vi "Get-date-string.vi"() -> (3 "Date string":string)   [LabVIEW 2013, in "HardwareCharacterization.lvlib" / "HC-Main.lvclass"]
uses:
  HC-Main.lvclass
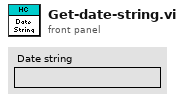
[diagram p1: front panel]
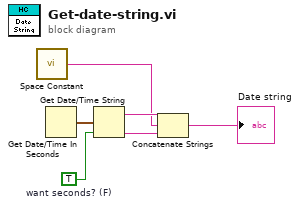
[diagram p0: block diagram]
diagram:
  w1 = TRUE  # want seconds? (F)
  n1 = call <vilib>:"Space Constant.vi"() -> ("String"=w2:string)
  n2 = Get Date/Time In Seconds() -> (seconds since 1Jan1904=w4:timestamp)
  n3 = Get Date/Time String(seconds (now)=w4, want seconds? (F)=w1) -> (date string=w5:string, time string=w3:string)  [unwired: 1 in]
  n4 = Concatenate Strings(w5, w2, w3) -> (→"Date string":string)
